vi "Signal Number Control.vi"(10 "Previous PMT1":bool, 11 "PMT1_signal in":u16) -> (2 "IO Module\\PMT1":bool, 3 "PMT1_signal out":u16)   [LabVIEW 2015]
uses:
  <vilib>/rvi/eio/common/nirviEmuTemplateMethod_errors.vi
  <vilib>/eio/EIONode/EIONode.xnode
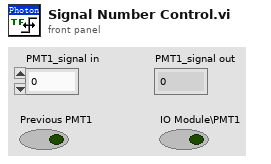
[diagram p1: front panel]
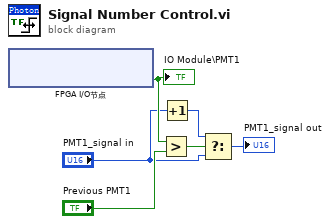
[diagram p0: block diagram]
diagram:
  n1 = xnode "FPGA I/O节点"() -> ("IO Module\\PMT1"=w6:bool)  [unwired: 1 in, 1 out]
  "IO Module\\PMT1" <- w6
  n2 = Greater?(x=w6, y="Previous PMT1") -> (0:w5:bool)
  n3 = Increment(x="PMT1_signal in") -> (x+1=w2:u16)
  n4 = Select(t=w2, s=w5, f="PMT1_signal in") -> (s? t:f=→"PMT1_signal out":u16)
